vi "Do i measure this quad.vi"(11 "Cell details":T1={"Measure?"=TRUE, "Area (cm^2)"=0.0, "Cell Label"="", "Cell Description"="", "Cell Position"=0, "Time in rig (s)"=0.0, "Time to next scan (s)"=0.0, "Scan number"=0.0, "When did you stick it in?"=0.0, "Time between scans (s)"=0.0, "Time of the last scan (s)"=0.0, "Scan settings in queue"=0, "Sample Holder"=0.0, "User Name"=""} {"Scan settings in queue" items=["Regular", "Inverted", "MartinaSettings"]; "Time of the last scan (s)" format="%<%H:%M:%S>t"; "When did you stick it in?" format="%<%H:%M:%S>t"; "Time to next scan (s)" format="%<%H:%M:%S>t"; "Time in rig (s)" format="%<%H:%M:%S>t"}) -> (3 "Measure cell?":bool)   [LabVIEW 2011]
uses:
  Typedefs/Queue cluster.ctl
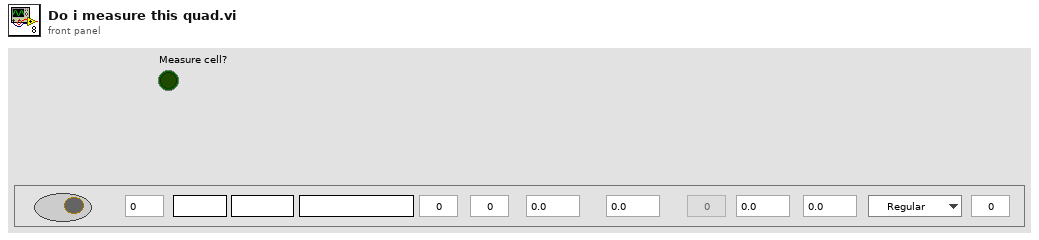
[diagram p1: front panel]
types:
  T1 = typedef "Queue cluster.ctl" = cluster{"Measure?":bool, "Area (cm^2)":dbl, "Cell Label":string, "Cell Description":string, "Cell Position":i32, "Time in rig (s)":dbl, "Time to next scan (s)":dbl, "Scan number":dbl, "When did you stick it in?":dbl, "Time between scans (s)":dbl, "Time of the last scan (s)":dbl, "Scan settings in queue":u16, "Sample Holder":dbl, "User Name":string}
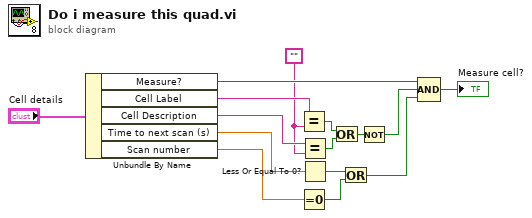
[diagram p0: block diagram]
diagram:
  w7 = ""
  n1 = Unbundle By Name("Cell details") -> ("Measure?"=w14:bool, "Cell Label"=w13:string, "Cell Description"=w12:string, "Time to next scan (s)"=w6:dbl, "Scan number"=w2:dbl)
  n2 = Equal?(x=w13, y=w7) -> (x = y?=w11:bool)
  n3 = Equal To 0?(x=w2) -> (x = 0?=w3:bool)
  n4 = Equal?(x=w12, y=w7) -> (x = y?=w10:bool)
  n5 = Less Or Equal To 0?(x=w6) -> (x <= 0?=w4:bool)
  n6 = Or(x=w11, y=w10) -> (x .or. y?=w9:bool)
  n7 = Or(x=w4, y=w3) -> (x .or. y?=w1:bool)
  n8 = Not(x=w9) -> (.not. x?=w8:bool)
  n9 = Compound Arithmetic op=AND(w14, w8, w1) -> (→"Measure cell?":bool)
